vi "Create Icon.vi"(11 "settings":T1) -> (3 "new picture":picture)   [LabVIEW 2017]
doc: "Creates new icon based on <b>settings</b>."
uses:
  CTLs/Settings.ctl
  CTLs/Template Frame.ctl
  CTLs/Text Format.ctl
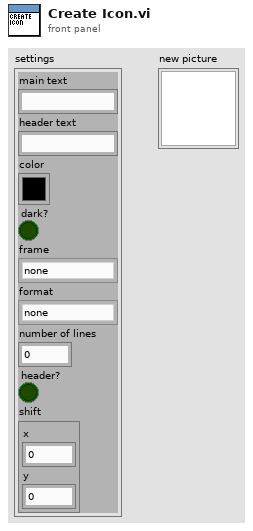
[diagram p1: front panel]
types:
  T1 = typedef "Settings.ctl" = cluster{"main text":string, "header text":string, "color":u32, "dark?":bool, "frame":T2, "format":T3, "number of lines":i32, "header?":bool, "shift":cluster{"x":i16, "y":i16}}
  T2 = typedef "Template Frame.ctl" = enum16{"none", "compact lib"}
  T3 = typedef "Text Format.ctl" = enum16{"none"}
  T4 = typedef "imagedata.ctl" = cluster{"image type":i32, "image depth":i32, "image":u8[], "mask":u8[], "colors":u32[], "Rectangle":cluster{"left":i16, "top":i16, "right":i16, "bottom":i16}}
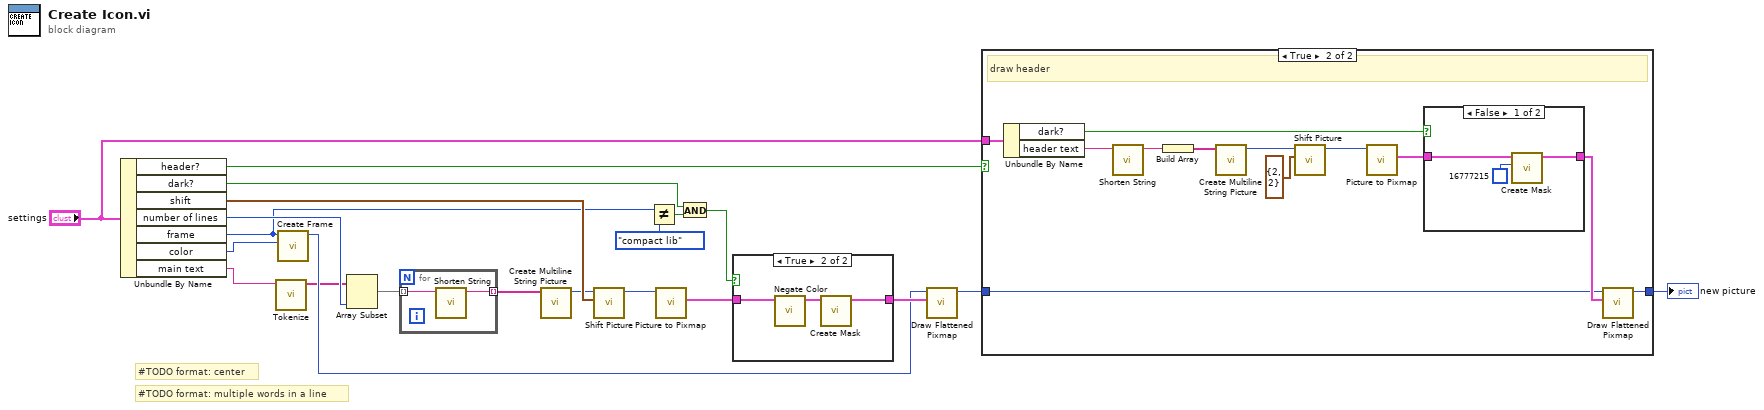
[diagram p0: block diagram]
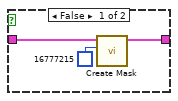
[diagram p2: hidden frame]
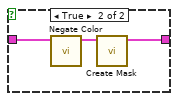
[diagram p4: hidden frame]
diagram:
  # "#TODO format: multiple words in a line"
  # "#TODO format: center"
  n1 = Unbundle By Name("settings") -> ("header?"=w12:bool, "dark?"=w2:bool, "shift"=w17:cluster{"x":i16, "y":i16}, "number of lines"=w15:i32, "frame"=w5:T2, "color"=w13:u32, "main text"=w6:string)
  n2 = call "Tokenize.vi"("string"=w6) -> ("tokens"=w14:string[])  [unwired: 10 in]
  n3 = call "Create Frame.vi"("color"=w13, "frame"=w5) -> ("frame picture"=w20:picture)  [unwired: 9 in]
  n4 = Array Subset(array=w14, length=w15) -> (w10:string[])  [unwired: 1 in]
  n5 = for {
    tunnel: w10 -> [w23] mode=indexing
    tunnel: [w22] -> w9 mode=indexing
    n6 = call "Shorten String.vi"("string in"=w23) -> ("string out"=w22:string)  [unwired: 10 in]
  }
  n7 = call "Create Multiline String Picture.vi"("array of strings"=w9) -> ("string picture"=w16:picture)  [unwired: 10 in]
  n8 = call "Shift Picture.vi"("shift"=w17, "picture in"=w16) -> ("picture out"=w18:picture)  [unwired: 9 in]
  n9 = Not Equal?(x=w5, y=Template_Frame."compact lib") -> (x != y?=w3:bool)
  n10 = call <vilib>:"Picture to Pixmap.vi"("picture"=w18) -> ("image data"=w19:T4)  [unwired: 9 in, 1 out]
  n11 = And(x=w2, y=w3) -> (x .and. y?=w1:bool)
  n12 = case shown="True" w1 {
    tunnel: w19 -> [w26 w29]
    tunnel: [w24 w27] -> w21
    frame False {
      n13 = call <vilib>:"Create Mask.vi"("Mask Color (Black)"=u32 16777215, "image data"=w26) -> ("image data"=w24:T4)  [unwired: 9 in]
    }
    frame True {
      n14 = call "Negate Color.vi"("image data in"=w29) -> ("image data out"=w28:T4)  [unwired: 10 in]
      n15 = call <vilib>:"Create Mask.vi"("image data"=w28) -> ("image data"=w27:T4)  [unwired: 10 in]
    }
  }
  n16 = call <vilib>:"Draw Flattened Pixmap.vi"("image data"=w21, "picture"=w20) -> ("new picture"=w8:picture)  [unwired: 7 in]
  n17 = case shown="True" w12 {
    tunnel: "settings" -> [_ w42]
    tunnel: w8 -> [w30 w32]
    tunnel: [w30 w31] -> w7
    frame False {
    }
    frame True {
      # "draw header"
      n18 = Unbundle By Name(w42) -> ("dark?"=w34:bool, "header text"=w41:string)
      n19 = call "Shorten String.vi"("string in"=w41) -> ("string out"=w40:string)  [unwired: 10 in]
      n20 = Build Array(w40) -> (w39:string[])
      n21 = call "Create Multiline String Picture.vi"("array of strings"=w39) -> ("string picture"=w38:picture)  [unwired: 10 in]
      n22 = call "Shift Picture.vi"("shift"=cluster{"x":i16, "y":i16} {"x"=2, "y"=2}, "picture in"=w38) -> ("picture out"=w33:picture)  [unwired: 9 in]
      n23 = call <vilib>:"Picture to Pixmap.vi"("picture"=w33) -> ("image data"=w36:T4)  [unwired: 9 in, 1 out]
      n24 = case shown="False" w34 {
        tunnel: w36 -> [w45 w48]
        tunnel: [w43 w46] -> w35
        frame False {
          n25 = call <vilib>:"Create Mask.vi"("Mask Color (Black)"=u32 16777215, "image data"=w45) -> ("image data"=w43:T4)  [unwired: 9 in]
        }
        frame True {
          n26 = call "Negate Color.vi"("image data in"=w48) -> ("image data out"=w47:T4)  [unwired: 10 in]
          n27 = call <vilib>:"Create Mask.vi"("image data"=w47) -> ("image data"=w46:T4)  [unwired: 10 in]
        }
      }
      n28 = call <vilib>:"Draw Flattened Pixmap.vi"("image data"=w35, "picture"=w32) -> ("new picture"=w31:picture)  [unwired: 7 in]
    }
  }
  "new picture" <- w7
